vi "calibration_to_vector.vi"(11 "Calibration in":T1 {"r bias" format="%_3p"; "Ks" format="%#_3p"}) -> (3 "State vector":dbl[](array[numeric]))   [LabVIEW 2026]
uses:
  calibration.ctl
  mag_globals.vi
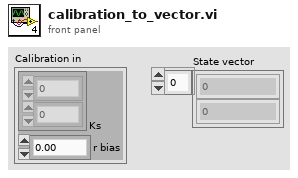
[diagram p1: front panel]
types:
  T1 = typedef "calibration.ctl" = cluster{"Ks":dbl[], "r bias":dbl}
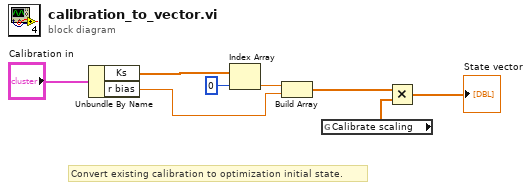
[diagram p0: block diagram]
diagram:
  # "Convert existing calibration to optimization initial state."
  n1 = Unbundle By Name("Calibration in") -> ("Ks"=w5:dbl[], "r bias"=w2:dbl)
  n2 = Index Array(array=w5, index=0 ("index (row)")) -> (element=w3:dbl)
  n3 = Build Array(w3, w2) -> (w1:dbl[])
  n4 = global read "mag_globals.vi" "Calibrate scaling"() -> (w8:dbl[])
  n5 = Multiply(x=w1, y=w8) -> (x*y=→"State vector":dbl[])
